vi "TapeModuleAssembly.vi"() -> ()   [LabVIEW 2021]
uses:
  <vilib>/Utility/error.llb/DialogType.ctl
  <vilib>/Utility/Data Type/NI_Data Type.lvlib
panel:
  in  "PressureSiPCB2":dbl[](array[numeric])=[35.0, 30.0, 0.0, 0.0]
  in  "GlPatternPCB2":path=path "C:/Users/TTUHEP/Documents/LabVIEW/Data/Patterns/SH_V3_Hybrid_SitoHex_2ndNov2023_rotatedminus240_Z12mm_Stage2.ngc"
  in  "GlPatternSi":path=path "C:/Users/TTUHEP/Documents/LabVIEW/Data/Patterns/Final_Patern/PCB_base_10-03-2022_2layers_1hexRestHorizontalwithCenterLine_ExtendedLines_SnakePattern_24F_ZsameAsLines_Combined.ngc"
  in  "GlPatternPCB1":path=path "C:/Users/TTUHEP/Documents/LabVIEW/Data/Patterns/SH_V3_Hybrid_SitoHex_2ndNov2023_rotatedminus240_Z12mm_Stage1.ngc"
  in  "PressureBPSi2":dbl[](array[numeric])=[30.0, 30.0, 18.0, 0.0]
  in  "PressureSiPCB1":dbl[](array[numeric])=[35.0, 30.0, 0.0, 0.0]
  in  "PressureBPSi1":dbl[](array[numeric])=[30.0, 30.0, 18.0, 0.0]
  in  "Glue2":bool=TRUE
  in  "Glue1":bool=TRUE
  in  "Operations 2":T1={"GoToTool"=TRUE, "PickTool"=TRUE, "GoToHB"=TRUE, "PickHB"=TRUE, "GoToSi"=TRUE, "PickSi"=TRUE, "GoToBP"=TRUE, "DropTool"=TRUE}
  in  "Operations":T1={"GoToTool"=TRUE, "PickTool"=TRUE, "GoToHB"=TRUE, "PickHB"=TRUE, "GoToSi"=TRUE, "PickSi"=TRUE, "GoToBP"=TRUE, "DropTool"=TRUE}
  in  "Position2":bool=TRUE
  in  "Position1":bool=TRUE
  in  "GoHome":bool
  in  "GlueVISA":refnum<visa-resource-name>="COM8"
  out "CurrentGlueCommand":string
  out "LogFile1":string
  out "LogFile2":string
  out "Log0":string
  out "Log2":string
  out "Log1":string
  out "Enter comment if any, and\npress \"Done\" at the end!!!":bool
  in  "Comment":string
  in  "Done":bool
  out "Error Out":errorcluster
  in  "Error In":errorcluster
  in  "Zone":enum16{"ZoneA", "ZoneB", "ZoneC", "ZoneD"}(ring)
  in  "AssmbType":enum16{"BothSiHB", "Sensor", "HB"}(ring)=enum."HB"
  in  "Initialize":T2={"Operator"="Sonaina", "ModuleName1"="", "ModuleName2"="", "SensorType"="", "SensorID1"="", "SensorID2"="", "BasePlateVersion"="", "PCBVersion"="", "NameOnPCB1"="", "NameOnPCB2"="", "GlueCartridge"="", "Temperature(F)"="", "RelHumidity(%)"=""}
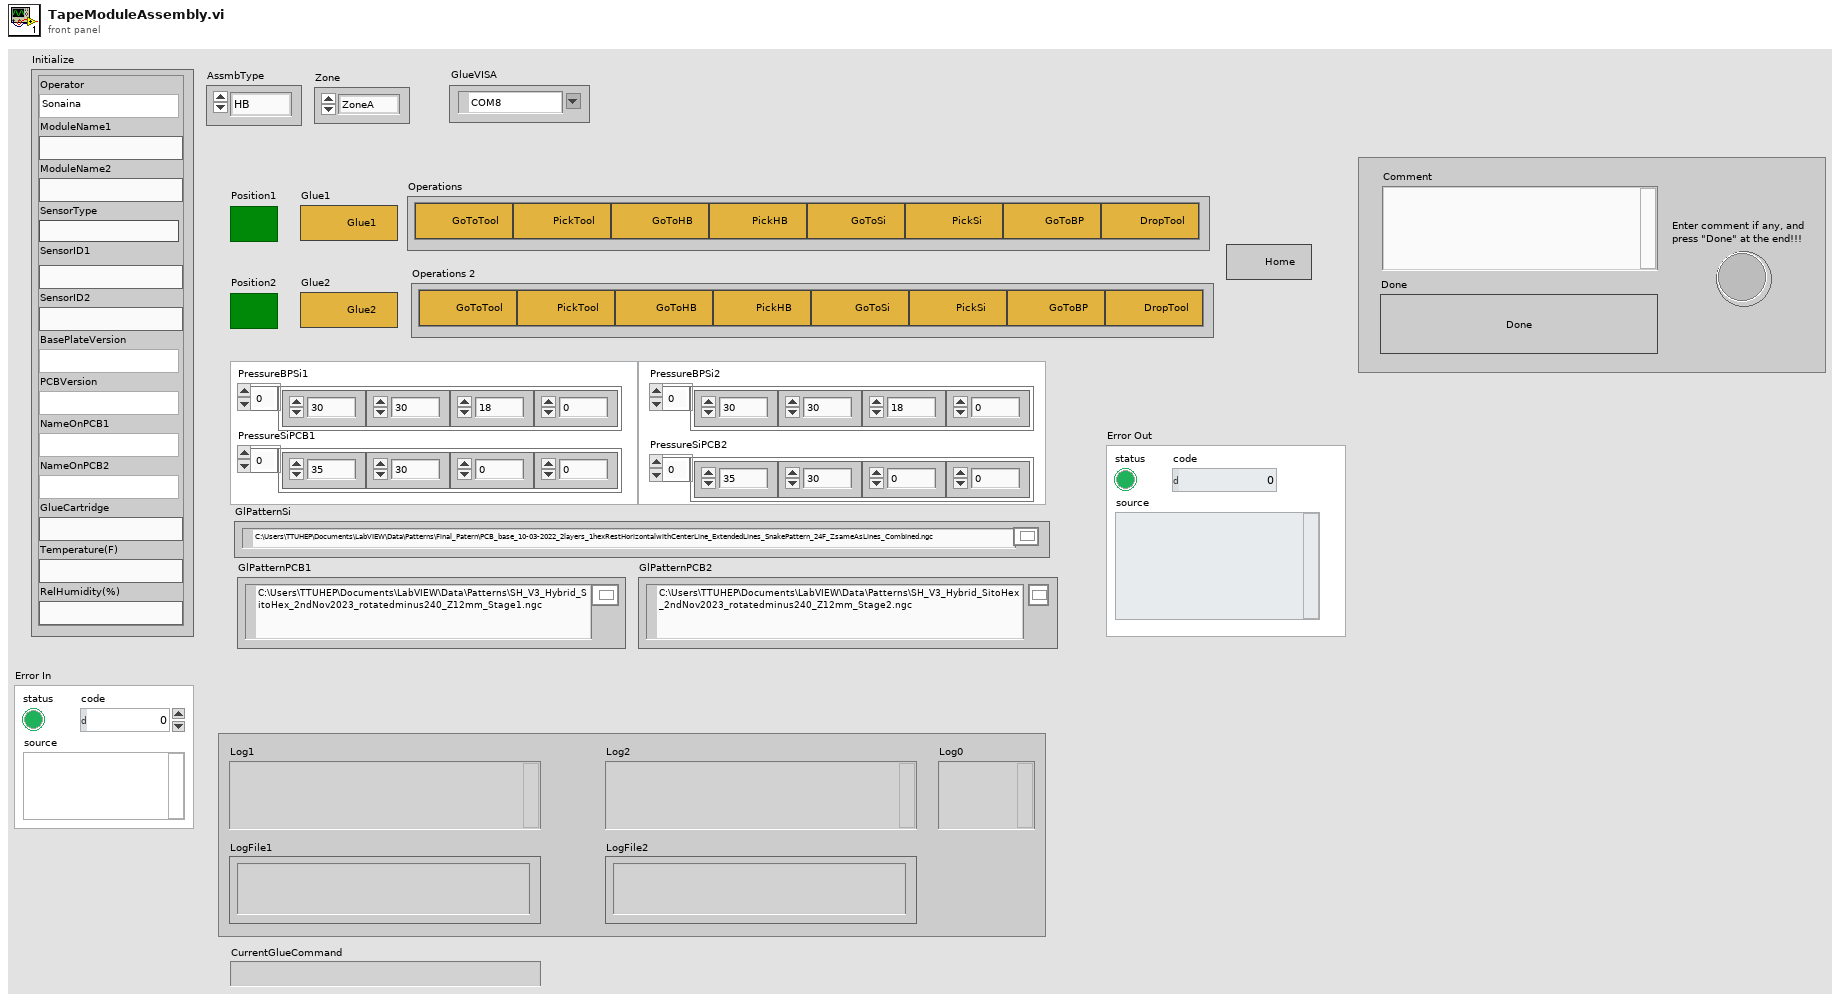
[diagram p1: front panel]
types:
  T1 = cluster{"GoToTool":bool, "PickTool":bool, "GoToHB":bool, "PickHB":bool, "GoToSi":bool, "PickSi":bool, "GoToBP":bool, "DropTool":bool}
  T2 = cluster{"Operator":string, "ModuleName1":string, "ModuleName2":string, "SensorType":string, "SensorID1":string, "SensorID2":string, "BasePlateVersion":string, "PCBVersion":string, "NameOnPCB1":string, "NameOnPCB2":string, "GlueCartridge":string, "Temperature(F)":string, "RelHumidity(%)":string}
  T3 = enum16{"open", "replace", "create", "open or create", "replace or create", "replace or create with confirmation"}
  T4 = typedef "DialogType.ctl" = u16
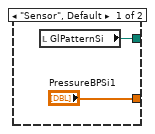
[diagram p5: hidden frame]
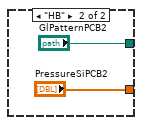
[diagram p8: hidden frame]
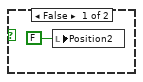
[diagram p11: hidden frame]
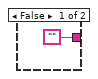
[diagram p14: hidden frame]
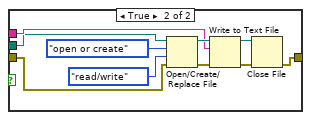
[diagram p16: hidden frame]
diagram:
  n1 = flat-sequence {
    tunnel: "Error In" -> [w23]
    tunnel: [w20] -> w9
    tunnel: w9 -> [w66]
    tunnel: [w67] -> w8
    tunnel: [w76] -> w14
    tunnel: w8 -> [w76]
    tunnel: [w68] -> w7
    tunnel: w14 -> [w86]
    tunnel: w7 -> [w83]
    tunnel: [w79] -> w6
    tunnel: w6 -> [w112]
    tunnel: [w110] -> w2
    tunnel: [w109] -> w1
    tunnel: [w168] -> w5
    tunnel: [w164] -> w3
    tunnel: w2 -> [w164]
    tunnel: w1 -> [w168]
    tunnel: w5 -> [w173]
    tunnel: [w177] -> w4
    tunnel: w3 -> [w176]
    tunnel: w4 -> [w231]
    tunnel: [w229] -> w17
    tunnel: w17 -> [w244]
    tunnel: [w244] -> w16
    tunnel: w16 -> [w251]
    tunnel: [w250] -> w18
    tunnel: w18 -> [w264]
    tunnel: [w265] -> w15
    tunnel: w15 -> [w275]
    tunnel: [w275] -> w10
    tunnel: [w280] -> w13
    tunnel: [w279] -> w11
    tunnel: w10 -> [w279]
    tunnel: w13 -> [w305]
    tunnel: [w293] -> w12
    tunnel: w11 -> [w295]
    frame #0 {
      w30 = "C:\\Users\\TTUHEP\\Documents\\LabVIEW\\GantryPrograms\\LogFiles\\" ("string")
      n2 = Unbundle By Name("Initialize") -> ("ModuleName1"=w35:string, "ModuleName2"=w36:string)
      n3 = Format Into String(format string="%s", "AssmbType") -> (resulting string=w33:string)  [unwired: 2 in, 1 out]
      n4 = Equal?(x=w35, y=w36) -> (x = y?=w32:bool)
      n5 = Concatenate Strings("_Assembly_" ("string"), w33, "_log.txt" ("string")) -> (w37:string)
      n6 = call "AddError.vi"("NoErrorMessage"="OK", "ErrorMessage"="ModuleName1 & 2 are the same.\nChoose different names.", "error in"=w23, "code"=-997, "Error?"=w32) -> ("Error out"=w22:errorcluster)  [unwired: 6 in]
      n7 = Concatenate Strings(w30, w35, w37) -> (w38:string)
      n8 = Concatenate Strings(w30, w36, w37) -> (w40:string)
      n9 = case shown="True" "Position1" {
        tunnel: w38 -> [_ w54]
        tunnel: w22 -> [w53 w57]
        tunnel: [w53 w55] -> w21
        frame False {
        }
        frame True {
          n10 = String To Path(string=w54) -> (path=w63:path)
          n11 = Concatenate Strings("This file exists. Choose a different file name." ("ErrorMessage"), w54) -> (w58:string)
          n12 = call <vilib>:"Check if File or Folder Exists.vi"("error in (no error)"=w57, "path"=w63) -> ("error out"=w56:errorcluster, "file or folder exists?"=w61:bool)  [unwired: 7 in, 1 out]
          n13 = call "AddError.vi"("NoErrorMessage"="P1FileOK", "ErrorMessage"=w58, "error in"=w56, "code"=-997, "Error?"=w61) -> ("Error out"=w55:errorcluster)  [unwired: 6 in]
          "LogFile1" <- w54
        }
      }
      n14 = case shown="True" "Position2" {
        tunnel: w40 -> [_ w43]
        tunnel: w21 -> [w42 w46]
        tunnel: [w42 w44] -> w20
        frame False {
        }
        frame True {
          n15 = String To Path(string=w43) -> (path=w52:path)
          n16 = Concatenate Strings("This file exists. Choose a different file name." ("ErrorMessage"), w43) -> (w47:string)
          n17 = call <vilib>:"Check if File or Folder Exists.vi"("error in (no error)"=w46, "path"=w52) -> ("error out"=w45:errorcluster, "file or folder exists?"=w50:bool)  [unwired: 7 in, 1 out]
          n18 = call "AddError.vi"("NoErrorMessage"="P2FileOK", "ErrorMessage"=w47, "error in"=w45, "code"=-997, "Error?"=w50) -> ("Error out"=w44:errorcluster)  [unwired: 6 in]
          "LogFile2" <- w43
        }
      }
    }
    frame #1 {
      w64 = T4 1 items=["no dialog", "OK message", "continue or stop message", "OK message + warnings", "continue/stop + warnings"] ("type of dialog (OK msg:1)")
      n19 = local write "Error Out"(w66) -> ()
      n20 = call <vilib>:"Simple Error Handler.vi"("type of dialog (OK msg:1)"=w64, "error in (no error)"=w66) -> ("error?"=w65:bool, "error out"=w67:errorcluster)  [unwired: 3 in, 3 out]
      n21 = Stop(stop? (T)=w65) -> ()
    }
    frame #2 {
      n22 = Get Date/Time String(date format (0)=enum16{"short", "long", "abbreviated"}."long", want seconds? (F)=TRUE) -> (date string=w74:string, time string=w75:string)  [unwired: 1 in]
      n23 = Concatenate Strings("StartDateTime: " ("string"), w74, ", ", w75, "\r\n") -> (w68:string)
      "Log0" <- w68
    }
    frame #3 {
      n24 = property on="Initialize" class="Clust (strict)"() -> ("Controls[]"=w89:refnum<vi>[])  [unwired: 2 in, 2 out]
      n25 = for {
        tunnel: w89 -> [w97] mode=indexing
        tunnel: [w93] -> w87 mode=indexing
        tunnel: [w92] -> w88 mode=indexing
        tunnel: w86 -> [w91]
        n26 = property class="Ctl"(reference=w97, error in=w91) -> (error out=w90:errorcluster, "ClassName"=w96:string, "Value"=w95:variant)  [unwired: 1 out]
        n27 = case shown="\"String\", Default" w96 {
          tunnel: w95 -> [w103]
          tunnel: [w100] -> w94
          tunnel: [w99] -> w93
          tunnel: w90 -> [w98]
          frame "String", Default {
            w104 = ": " ("string")
            n28 = call <vilib>:"Get Type Information.vi"("error in (no error)"=w98, "variant"=w103) -> ("error out"=w101:errorcluster, "name"=w102:string)  [unwired: 5 in, 3 out]
            n29 = Variant To Data(error in=w101, type=w104, Variant=w103) -> (data=w105:string, error out=w99:errorcluster)
            n30 = Concatenate Strings(w102, w104, w105, "\r\n") -> (w100:string)
          }
        }
        n31 = Build Array(w94) -> (w92:string[])
      }
      n32 = Concatenate Strings(w83, w88) -> (w84:string)
      "Log1" <- w84
      "Log2" <- w84
      n33 = Merge Errors(w87) -> (w85:errorcluster)
      n34 = local write "Log0"(w84) -> ()
      n35 = call "Connect.vi"("error in (no error)"=w85) -> ("error out"=w81:errorcluster, "controller"=w82:refnum<k24>)  [unwired: 9 in]
      n36 = call "ExecuteCommand.vi"("error in (no error)"=w81, "Command Code"="G90\nG1 Z0 F100", "controller in"=w82) -> ("error out"=w78:errorcluster, "controller out"=w77:refnum<k24>)  [unwired: 6 in, 1 out]
      n37 = call "Disconnect.vi"("error in (no error)"=w78, "controller"=w77) -> ("error out"=w79:errorcluster)  [unwired: 9 in]
    }
    frame #4 {
      w110 = path "C:/Users/TTUHEP/Documents/LabVIEW/GantryPrograms/Configs/DispensePressCorrection.txt" ("TextFile")
      n38 = local read "Position1"() -> (w116:bool)
      n39 = And(x="Glue1", y=w116) -> (x .and. y?=w114:bool)
      n40 = call "Connect.vi"("error in (no error)"=w112) -> ("error out"=w113:errorcluster, "controller"=w111:refnum<k24>)  [unwired: 9 in]
      n41 = case shown="True" w114 {
        tunnel: w111 -> [w118 w159]
        tunnel: w113 -> [w120 w135]
        tunnel: [w118 w121] -> w107
        tunnel: [w120 w157] -> w108
        tunnel: "GlueVISA" -> [w119 w155]
        tunnel: [w119 w155] -> _
        tunnel: w110 -> [_ w122]
        frame False {
        }
        frame True {
          n42 = local read "Zone"() -> (w137:enum16{"ZoneA", "ZoneB", "ZoneC", "ZoneD"})
          n43 = local read "AssmbType"() -> (w156:enum16{"BothSiHB", "Sensor", "HB"})
          n44 = call "GetSyringeXYZ.vi"("error in"=w135, "Position"=enum16{"1", "2"}."1", "Zone"=w137) -> ("Error out"=w133:errorcluster, "SyringeZ"=w132:dbl, "SyringeY"=w131:dbl, "SyringeX"=w134:dbl)  [unwired: 5 in]
          n45 = case shown="\"HB\"" w156 {
            tunnel: [w161 "GlPatternPCB1"] -> w154
            tunnel: ["PressureBPSi1" "PressureSiPCB1"] -> w124
            frame "Sensor", Default {
              n46 = local read "GlPatternSi"() -> (w161:path)
            }
            frame "HB" {
            }
          }
          n47 = call <vilib>:"Simple Error Handler.vi"("error in (no error)"=w133) -> ("error?"=w139:bool, "error out"=w126:errorcluster)  [unwired: 4 in, 3 out]
          n48 = Build Array(w134, w131, w132, 0.0 ("element")) -> (w146:dbl[])
          n49 = Stop(stop? (T)=w139) -> ()
          n50 = Array To Spreadsheet String(delimiter (Tab)=",", array=w146, 3:"%f" ("format string")) -> (spreadsheet string=w144:string)
          n51 = call "GetArrayFmTxtFile.vi"("error in"=w126, "LineNo."=0, "TextFile"=w122) -> ("error out"=w125:errorcluster, "Array"=w129:dbl[])
          n52 = Index Array(array=w129, index=0) -> (element=w127:dbl)
          n53 = Multiply(x=w124, y=w127) -> (x*y=w123:dbl[])
          n54 = call "Dispenser_v2.vi"("VISA resource name"=w155, "X"=w134, "Y"=w131, "controller in"=w159, "Path"=w154, "Pressure"=w123, "Z"=w132, "error in (no error)"=w125) -> ("Comm"=→"CurrentGlueCommand":string, "controller out"=w121:refnum<k24>, "error out"=w157:errorcluster)  [unwired: 3 in, 2 out]
          n55 = Array To Spreadsheet String(delimiter (Tab)=",", array=w123, 3:"%f" ("format string")) -> (spreadsheet string=w150:string)
          n56 = Path To String(path=w154) -> (string=w151:string)
          n57 = local read "Log0"() -> (w138:string)
          n58 = Concatenate Strings(w138, "GluePattern: ", w151, "\r\n", "GluePressure: ", w150, "Syringe_XYZU: ", w144) -> (w143:string)
          n59 = local write "Log1"(w143) -> ()
        }
      }
      n60 = call "Disconnect.vi"("error in (no error)"=w108, "controller"=w107) -> ("error out"=w109:errorcluster)  [unwired: 9 in]
    }
    frame #5 {
      n61 = local read "Position2"() -> (w165:bool)
      n62 = And(x="Glue2", y=w165) -> (x .and. y?=w167:bool)
      n63 = case shown="True" w167 {
        frame False {
        }
        frame True {
          n64 = Two Button Dialog(message="Glue on position2?", 1:"No" ("F button name (\"Cancel\")"), 2:"Yes" ("button name (\"OK\")")) -> (T button?=w169:bool)
          n65 = local write "Glue2"(w169) -> ()
        }
      }
    }
    frame #6 {
      n66 = local read "Position2"() -> (w181:bool)
      n67 = local read "Glue2"() -> (w183:bool)
      n68 = local read "GlueVISA"() -> (w180:refnum<visa-resource-name>)
      n69 = And(x=w183, y=w181) -> (x .and. y?=w182:bool)
      n70 = call "Connect.vi"("error in (no error)"=w173) -> ("error out"=w174:errorcluster, "controller"=w175:refnum<k24>)  [unwired: 9 in]
      n71 = case shown="True" w182 {
        tunnel: w175 -> [w185 w224]
        tunnel: w174 -> [w184 w199]
        tunnel: [w185 w223] -> w179
        tunnel: [w184 w222] -> w178
        tunnel: w180 -> [_ w221]
        tunnel: w176 -> [_ w186]
        frame False {
        }
        frame True {
          n72 = local read "Zone"() -> (w201:enum16{"ZoneA", "ZoneB", "ZoneC", "ZoneD"})
          n73 = local read "AssmbType"() -> (w220:enum16{"BothSiHB", "Sensor", "HB"})
          n74 = call "GetSyringeXYZ.vi"("error in"=w199, "Position"=enum16{"1", "2"}."2", "Zone"=w201) -> ("Error out"=w198:errorcluster, "SyringeZ"=w196:dbl, "SyringeY"=w195:dbl, "SyringeX"=w197:dbl)  [unwired: 5 in]
          n75 = case shown="\"Sensor\", Default" w220 {
            tunnel: ["PressureBPSi2" "PressureSiPCB2"] -> w190
            tunnel: [w226 "GlPatternPCB2"] -> w209
            frame "Sensor", Default {
              n76 = local read "GlPatternSi"() -> (w226:path)
            }
            frame "HB" {
            }
          }
          n77 = call <vilib>:"Simple Error Handler.vi"("error in (no error)"=w198) -> ("error?"=w202:bool, "error out"=w188:errorcluster)  [unwired: 4 in, 3 out]
          n78 = Build Array(w197, w195, w196, 0.0 ("element")) -> (w207:dbl[])
          n79 = Stop(stop? (T)=w202) -> ()
          n80 = Array To Spreadsheet String(delimiter (Tab)=",", array=w207, 3:"%f" ("format string")) -> (spreadsheet string=w213:string)
          n81 = call "GetArrayFmTxtFile.vi"("error in"=w188, "LineNo."=0, "TextFile"=w186) -> ("error out"=w187:errorcluster, "Array"=w193:dbl[])
          n82 = Index Array(array=w193, index=0) -> (element=w191:dbl)
          n83 = Multiply(x=w190, y=w191) -> (x*y=w189:dbl[])
          n84 = call "Dispenser_v2.vi"("VISA resource name"=w221, "X"=w197, "Y"=w195, "controller in"=w224, "Path"=w209, "Pressure"=w189, "Z"=w196, "error in (no error)"=w187) -> ("Comm"=w204:string, "controller out"=w223:refnum<k24>, "error out"=w222:errorcluster)  [unwired: 3 in, 2 out]
          n85 = Array To Spreadsheet String(delimiter (Tab)=",", array=w189, 3:"%f" ("format string")) -> (spreadsheet string=w208:string)
          n86 = local write "CurrentGlueCommand"(w204) -> ()
          n87 = Path To String(path=w209) -> (string=w217:string)
          n88 = local read "Log0"() -> (w203:string)
          n89 = Concatenate Strings(w203, "GluePattern: ", w217, "\r\n", "GluePressure: ", w208, "Syringe_XYZU: ", w213) -> (w205:string)
          n90 = local write "Log2"(w205) -> ()
        }
      }
      n91 = call "Disconnect.vi"("error in (no error)"=w178, "controller"=w179) -> ("error out"=w177:errorcluster)  [unwired: 9 in]
    }
    frame #7 {
      n92 = local read "Position1"() -> (w230:bool)
      n93 = case shown="True" w230 {
        tunnel: w231 -> [w232 w239]
        tunnel: [w232 w242] -> w229
        frame False {
        }
        frame True {
          n94 = local read "AssmbType"() -> (w233:enum16{"BothSiHB", "Sensor", "HB"})
          n95 = local read "Zone"() -> (w240:enum16{"ZoneA", "ZoneB", "ZoneC", "ZoneD"})
          n96 = call "PickAndPlace_SiAndHB.vi"("Operations"="Operations", "VacuumStates"=path "C:/Users/TTUHEP/Documents/LabVIEW/GantryPrograms/Configs/PickPlaceVacuumStates.json", "AssmbType"=w233, "Zone"=w240, "Position"=enum16{"1", "2"}."1", "Error In"=w239) -> ("Log"=w236:string, "Error Out"=w242:errorcluster)  [unwired: 8 in]
          n97 = local read "Log1"() -> (w237:string)
          n98 = Concatenate Strings(w237, w236) -> (w238:string)
          n99 = local write "Log1"(w238) -> ()
        }
      }
    }
    frame #8 {
      n100 = local read "Position2"() -> (w243:bool)
      n101 = case shown="True" w243 {
        frame False {
        }
        frame True {
          n102 = Two Button Dialog(message="Start pick and place in position 2?", 1:"No" ("F button name (\"Cancel\")"), 2:"Yes" ("button name (\"OK\")")) -> (T button?=w245:bool)
          n103 = case shown="True" w245 {
            frame False {
              n104 = local write "Position2"(FALSE ("Position2")) -> ()
            }
            frame True {
            }
          }
        }
      }
    }
    frame #9 {
      n105 = local read "Position2"() -> (w252:bool)
      n106 = case shown="True" w252 {
        tunnel: w251 -> [w253 w261]
        tunnel: [w253 w260] -> w250
        frame False {
        }
        frame True {
          n107 = local read "AssmbType"() -> (w254:enum16{"BothSiHB", "Sensor", "HB"})
          n108 = local read "Zone"() -> (w263:enum16{"ZoneA", "ZoneB", "ZoneC", "ZoneD"})
          n109 = call "PickAndPlace_SiAndHB.vi"("Operations"="Operations 2", "VacuumStates"=path "C:/Users/TTUHEP/Documents/LabVIEW/GantryPrograms/Configs/PickPlaceVacuumStates.json", "AssmbType"=w254, "Zone"=w263, "Position"=enum16{"1", "2"}."2", "Error In"=w261) -> ("Log"=w259:string, "Error Out"=w260:errorcluster)  [unwired: 8 in]
          n110 = local read "Log2"() -> (w258:string)
          n111 = Concatenate Strings(w258, w259) -> (w257:string)
          n112 = local write "Log2"(w257) -> ()
        }
      }
    }
    frame #10 {
      n113 = case shown="True" "GoHome" {
        tunnel: [w267 w268] -> w265
        tunnel: w264 -> [w267 w269]
        frame False {
        }
        frame True {
          n114 = call "Connect.vi"("error in (no error)"=w269) -> ("error out"=w274:errorcluster, "controller"=w271:refnum<k24>)  [unwired: 9 in]
          n115 = call "ExecuteCommand.vi"("error in (no error)"=w274, "Command Code"="G90\nG1 X0 Y0 Z0 F100", "controller in"=w271) -> ("error out"=w273:errorcluster, "controller out"=w270:refnum<k24>)  [unwired: 6 in, 1 out]
          n116 = call "Disconnect.vi"("error in (no error)"=w273, "controller"=w270) -> ("error out"=w268:errorcluster)  [unwired: 9 in]
        }
      }
    }
    frame #11 {
    }
    frame #12 {
      n117 = local read "Position1"() -> (w278:bool)
      n118 = local read "Position2"() -> (w277:bool)
      n119 = Or(x=w278, y=w277) -> (x .or. y?=w276:bool)
      n120 = case shown="True" w276 {
        tunnel: ["" w283] -> w280
        frame False {
        }
        frame True {
          n121 = while {
            tunnel: [w287] -> w283
            shift-right: [w285] -> _
            shift-left: TRUE -> [w286]
            stop <- "Done" stop-if-true
            n122 = Not(x=w286) -> (.not. x?=w285:bool)
            "Enter comment if any, and\npress \"Done\" at the end!!!" <- w285
            n123 = Wait (ms)(milliseconds to wait=u32 100) -> ()  [unwired: 1 out]
            n124 = Concatenate Strings("-------------\nComments:", "Comment") -> (w287:string)
          }
        }
      }
    }
    frame #13 {
      w298 = "\r\n"
      n125 = local write "Enter comment if any, and\npress \"Done\" at the end!!!"(FALSE ("Press Done at the end!!!")) -> ()
      n126 = Get Date/Time String(date format (0)=enum16{"short", "long", "abbreviated"}."long", want seconds? (F)=TRUE) -> (date string=w303:string, time string=w304:string)  [unwired: 1 in]
      n127 = local read "Position1"() -> (w292:bool)
      n128 = Build Array(w298, "EndDateTime: " ("string"), w303, ", ", w304, w298) -> (w297:string[])
      n129 = case shown="True" w292 {
        tunnel: w305 -> [_ w342]
        tunnel: w297 -> [_ w341]
        tunnel: w295 -> [w331 w339]
        tunnel: [w331 w338] -> w294
        frame False {
        }
        frame True {
          w343 = "\r\n"
          n130 = local read "Log1"() -> (w337:string)
          n131 = Concatenate Strings(w337, w343, w342, w343, w341) -> (w340:string)
          n132 = local write "Log1"(w340) -> ()
          n133 = local read "LogFile1"() -> (w333:string)
          n134 = Concatenate Strings("Write assembly log1 to file " ("string"), w333, "?" ("string")) -> (w334:string)
          n135 = Two Button Dialog(message=w334) -> (T button?=w332:bool)  [unwired: 2 in]
          n136 = case shown="True" w332 {
            tunnel: w340 -> [_ w349]
            tunnel: w339 -> [w344 w347]
            tunnel: [w344 w346] -> w338
            tunnel: w333 -> [_ w345]
            frame False {
            }
            frame True {
              n137 = String To Path(string=w345) -> (path=w348:path)
              n138 = Open/Create/Replace File(file path (use dialog)=w348, error in=w347, operation (0:open)=T3."open or create", access (0:read/write)=enum16{"read/write", "read-only", "write-only"}."read/write") -> (refnum out=w354:refnum<file>, error out=w353:errorcluster)  [unwired: 2 in, 1 out]
              n139 = Write to Text File(file (use dialog)=w354, text=w349, error in=w353) -> (refnum out=w355:refnum<file>, error out=w352:errorcluster)  [unwired: 1 in, 1 out]
              n140 = Close File(refnum=w355, error in=w352) -> (error out=w346:errorcluster)  [unwired: 1 out]
            }
          }
        }
      }
      n141 = local read "Position2"() -> (w291:bool)
      n142 = case shown="True" w291 {
        tunnel: w305 -> [_ w318]
        tunnel: w297 -> [_ w317]
        tunnel: w294 -> [w306 w315]
        tunnel: [w306 w314] -> w293
        frame False {
        }
        frame True {
          w319 = "\r\n"
          n143 = local read "Log2"() -> (w312:string)
          n144 = Concatenate Strings(w312, w319, w318, w319, w317) -> (w316:string)
          n145 = local write "Log2"(w316) -> ()
          n146 = local read "LogFile2"() -> (w308:string)
          n147 = String To Path(string=w308) -> (path=w313:path)
          n148 = Concatenate Strings("Write assembly log2 to file " ("string"), w308, "?" ("string")) -> (w311:string)
          n149 = Two Button Dialog(message=w311) -> (T button?=w307:bool)  [unwired: 2 in]
          n150 = case shown="False" w307 {
            tunnel: w316 -> [_ w324]
            tunnel: w315 -> [w320 w323]
            tunnel: [w320 w322] -> w314
            tunnel: w313 -> [_ w321]
            frame False {
            }
            frame True {
              n151 = Open/Create/Replace File(file path (use dialog)=w321, error in=w323, operation (0:open)=T3."open or create", access (0:read/write)=enum16{"read/write", "read-only", "write-only"}."read/write") -> (refnum out=w329:refnum<file>, error out=w328:errorcluster)  [unwired: 2 in, 1 out]
              n152 = Write to Text File(file (use dialog)=w329, text=w324, error in=w328) -> (refnum out=w330:refnum<file>, error out=w327:errorcluster)  [unwired: 1 in, 1 out]
              n153 = Close File(refnum=w330, error in=w327) -> (error out=w322:errorcluster)  [unwired: 1 out]
            }
          }
        }
      }
    }
  }
  "Error Out" <- w12
